vi "updatepos.vi"(8 "error in (no error)":errorcluster, 10 "Theta enabled":bool, 11 "VISA Refnum in":refnum<visa-resource-name>) -> (0 "error out":errorcluster, 2 "PosArray":dbl[](array[numeric]), 3 "VISA Refnum out":refnum<visa-resource-name>)   [LabVIEW 2020]
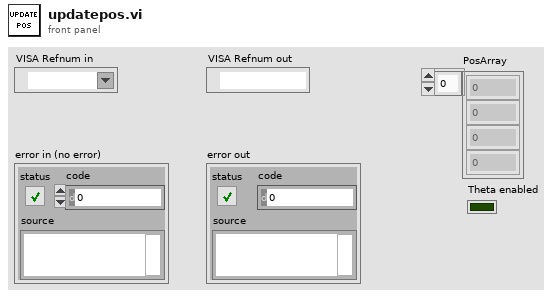
[diagram p1: front panel]
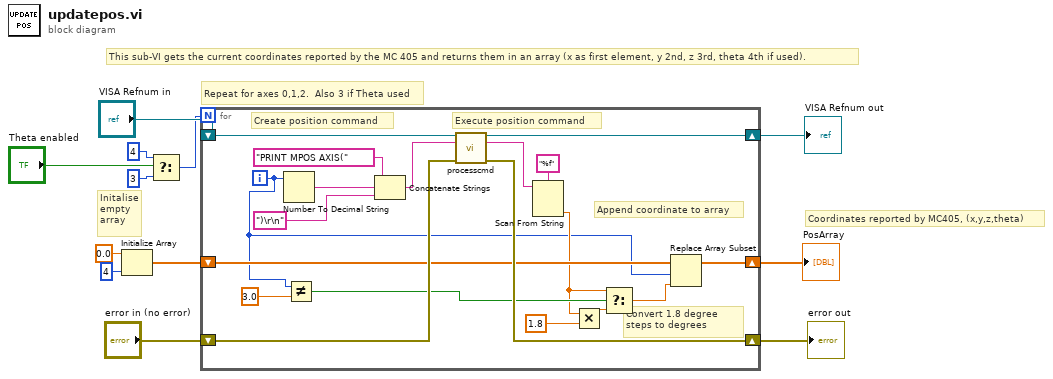
[diagram p0: block diagram]
diagram:
  # "This sub-VI gets the current coordinates reported by the MC 405 and returns them in an array (x as first element, y 2nd, z 3rd, theta 4th if used)."
  # "Initalise\nempty \narray"
  # "Coordinates reported by MC405, (x,y,z,theta)"
  # "Repeat for axes 0,1,2.  Also 3 if Theta used"
  n1 = Initialize Array(0.0 ("element"), 4 ("dimension size")) -> (w6:dbl[])
  n2 = Select(t=4, s="Theta enabled", f=3) -> (s? t:f=w4:i32)
  n3 = for {
    N: w4 -> [_]
    shift-right: [w31] -> w12
    shift-left: "VISA Refnum in" -> [w30]
    shift-right: [w29] -> w10
    shift-left: "error in (no error)" -> [w28]
    shift-right: [w20] -> w5
    shift-left: w6 -> [w21]
    i -> [w13]
    # "Convert 1.8 degree steps to degrees"
    # "Append coordinate to array"
    # "Execute position command"
    # "Create position command"
    n4 = Number To Decimal String(number=w13) -> (decimal integer string=w24:string)  [unwired: 1 in]
    n5 = Not Equal?(x=w13, y=3.0) -> (x != y?=w18:bool)
    n6 = Concatenate Strings("PRINT MPOS AXIS(" ("write buffer"), w24, ")\r\n" ("string")) -> (w22:string)
    n7 = call "processcmd.vi"("VISA Refnum in"=w30, "write buffer"=w22, "error in (no error)"=w28) -> ("VISA Refnum out"=w31:refnum<visa-resource-name>, "read buffer"=w27:string, "error out"=w29:errorcluster)  [unwired: 10 in]
    n8 = Scan From String(format string="%f", input string=w27) -> (output 1=w15:dbl)  [unwired: 3 in, 3 out]
    n9 = Multiply(x=w15, y=1.8) -> (x*y=w16:dbl)
    n10 = Select(t=w15, s=w18, f=w16) -> (s? t:f=w17:dbl)
    n11 = Replace Array Subset(array=w21, new element=w17, index=w13) -> (w20:dbl[])
  }
  "VISA Refnum out" <- w12
  "error out" <- w10
  "PosArray" <- w5
